vi "ClientAsig.vi"() -> ()   [LabVIEW 2021]
uses:
  <vilib>/Utility/file.llb/Write Delimited Spreadsheet (string).vi
panel:
  in  "login database":string[][](table)
  in  "Tab Control":T1(tab)
  in  "register":bool
  in  "login":bool
  in  "Password":string
  in  "Username":string
  in  "Front door":bool
  in  "On / off":bool
  in  "LR light 4":bool
  in  "LR light 3":bool
  in  "LR light 2":bool
  in  "LR light1":bool
  in  "LR curtain":dbl(knob) scale=0.0..100.0
  in  "aircorn temp":dbl(knob) scale=16.0..28.0
  in  "mb light 2":bool
  in  "mb light 1":bool
  in  "mb door":bool
  in  "bd light 1":bool
  in  "bd2 light 1":bool
  in  "bd2 light 2":bool
  in  "bd2 curtain 2":dbl(knob) scale=0.0..100.0
  in  "date&time":bool
  in  "balcony ct":dbl(knob) scale=0.0..100.0
  in  "balcony 1 light":bool
  in  "balcony light 1":bool
  in  "balcony light 2":bool
  in  "balcony light 3":bool
  in  "balcony1 ct":dbl(knob) scale=0.0..100.0
  in  "30 secs":bool
  in  "kc light 1":bool
  in  "kc light 2":bool
  in  "kc light 3":bool
  in  "Forward Button":bool
  in  "Back Button":bool
  in  "Pause Button":bool
  in  "mute":bool
  in  "volume":dbl(knob) scale=0.0..100.0
  in  "tv button3":bool
  in  "tv on":bool
  in  "tv off":bool
  in  "tv button 2":bool
  in  "tv button1":bool
  in  "forward":bool
  in  "back":bool
  in  "Refresh":bool
  in  "open":bool
  in  "website":string(combo)
  # "Welcome home"
  # "click other room to view other control"
  # "Living Room"
  # "lightning"
  # "aircorn"
  # "Curtain"
  # "master bedroom"
  # "lightning"
  # "door"
  # "bedroom 1"
  # "bedroom 2"
  # "lightning"
  # "curtain"
  # "balcony"
  # "lightning"
  # "curtain"
  # "Kitchen"
  # "timer"
  # "remote control TV"
  # "web broswer"
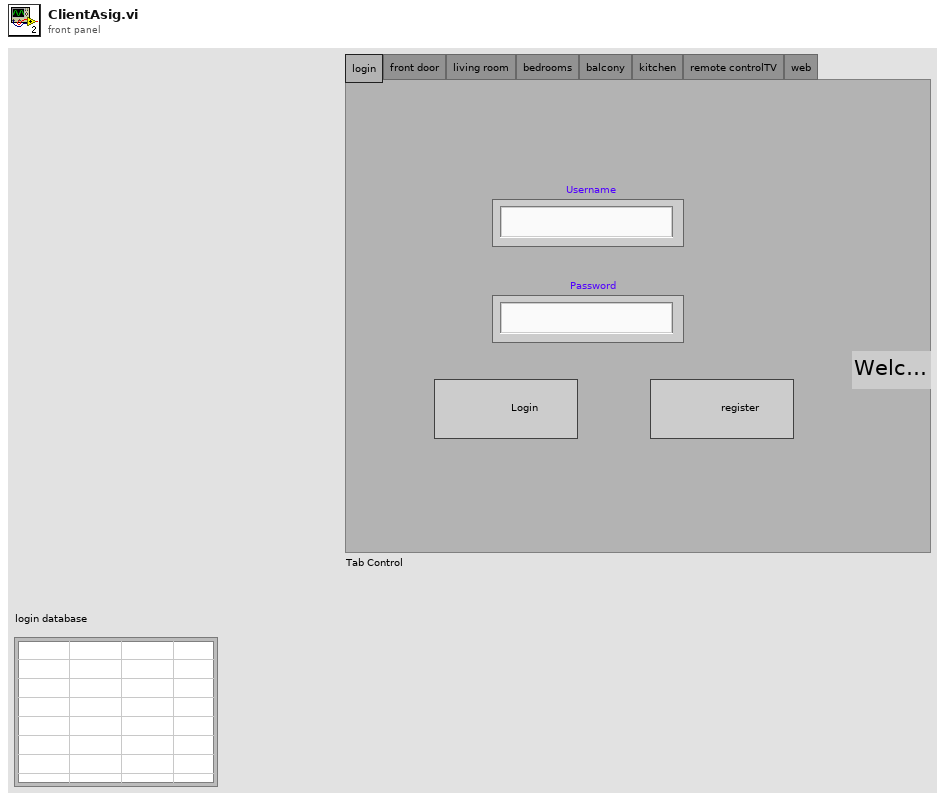
[diagram p1: front panel]
types:
  T1 = enum32{"login", "front door", "living room", "bedrooms", "balcony", "kitchen", "remote controlTV", "web"}
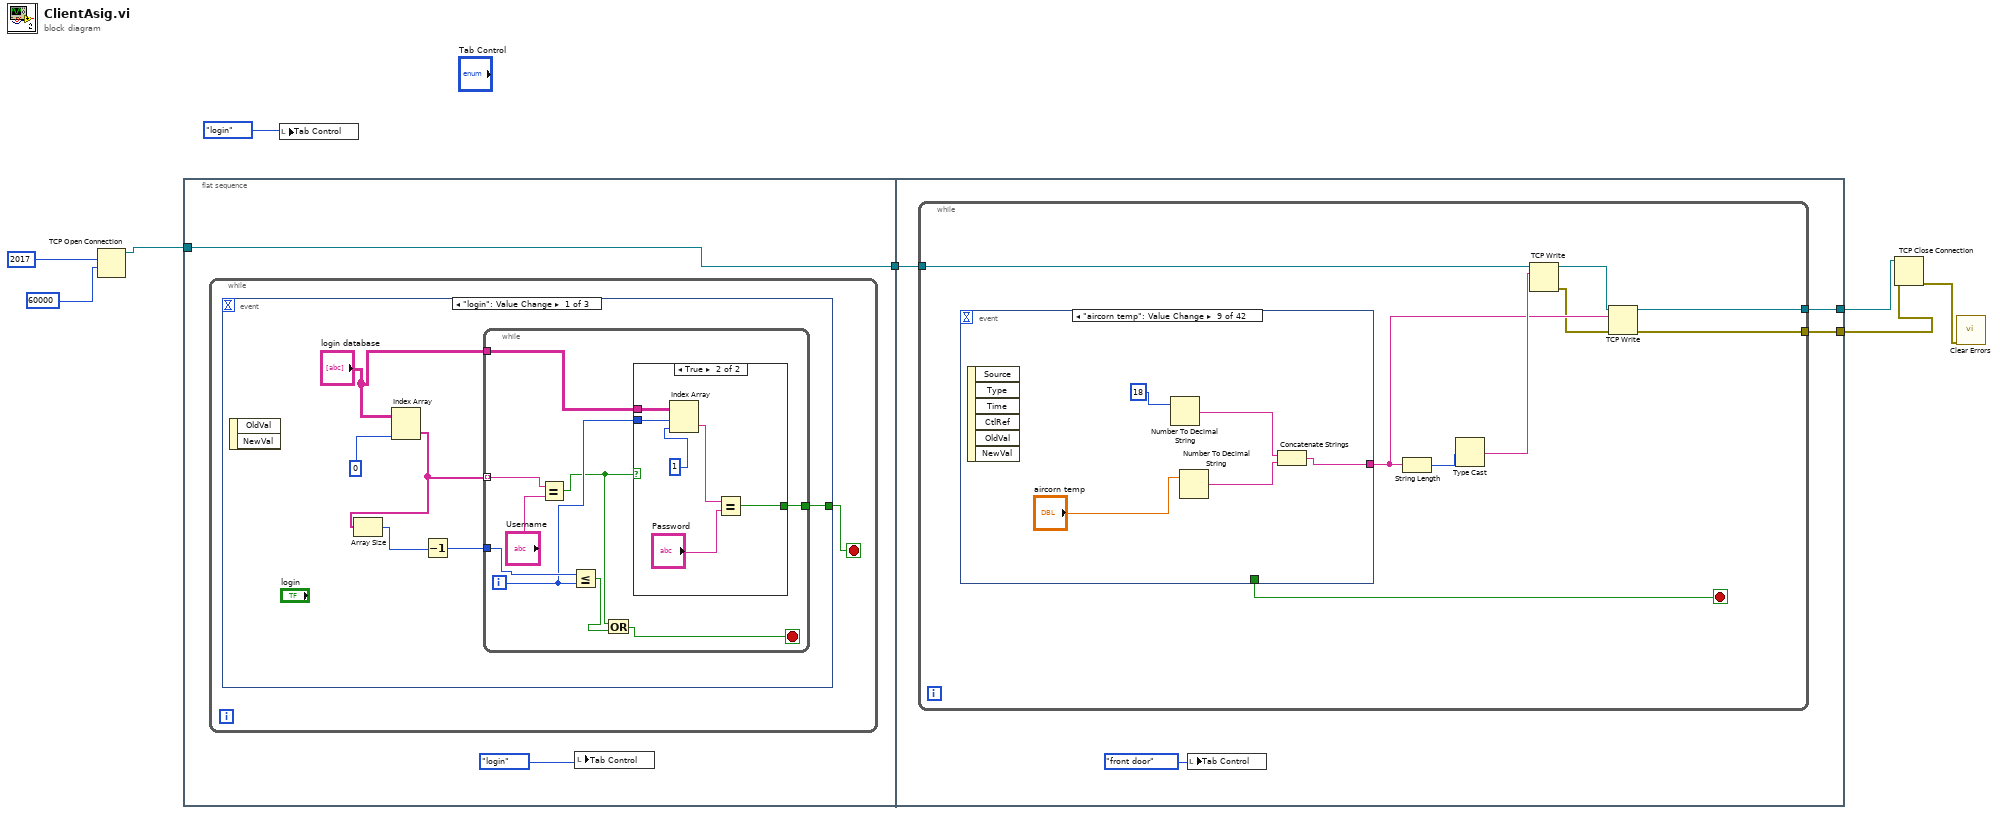
[diagram p0: block diagram]
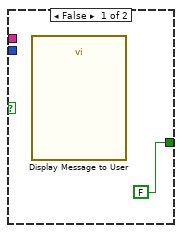
[diagram p2: hidden frame]
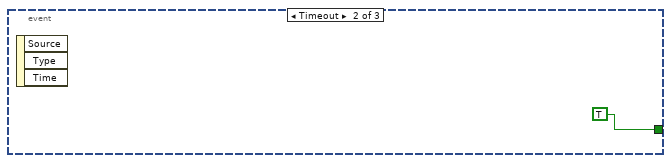
[diagram p3: hidden frame]
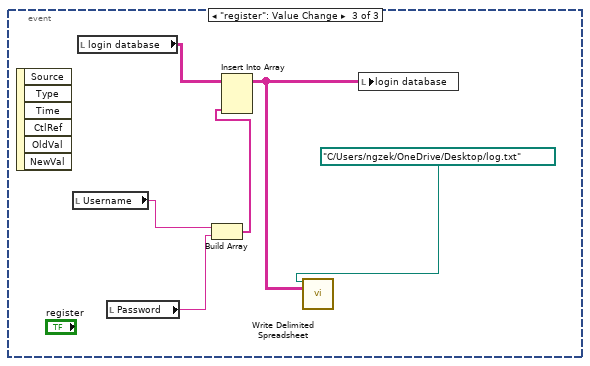
[diagram p4: hidden frame]
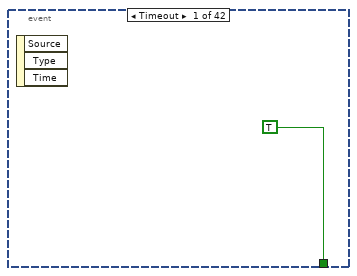
[diagram p5: hidden frame]
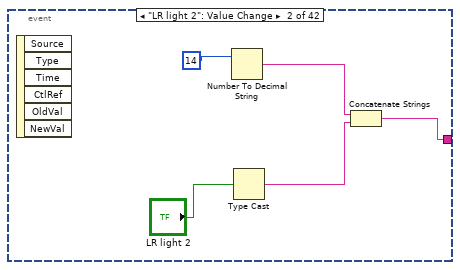
[diagram p6: hidden frame]
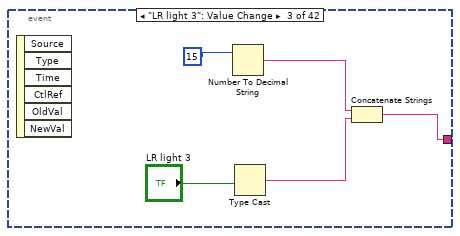
[diagram p7: hidden frame]
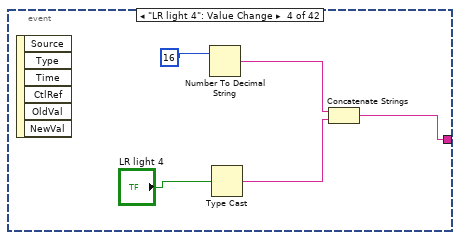
[diagram p8: hidden frame]
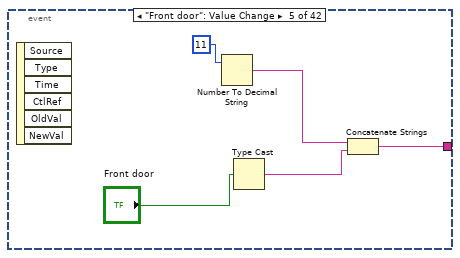
[diagram p9: hidden frame]
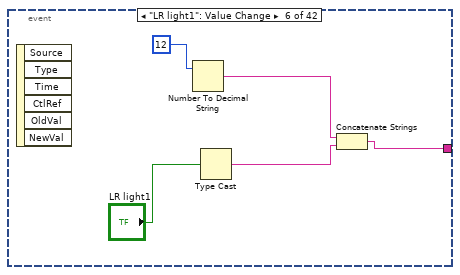
[diagram p10: hidden frame]
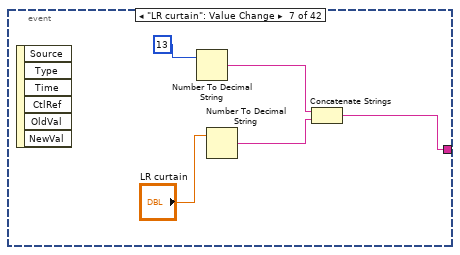
[diagram p11: hidden frame]
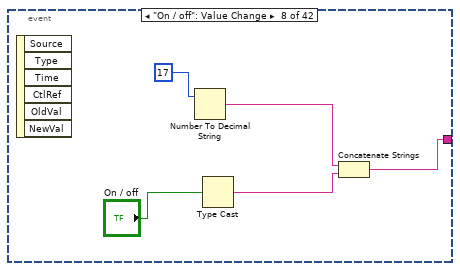
[diagram p12: hidden frame]
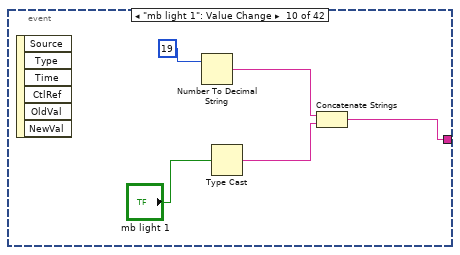
[diagram p13: hidden frame]
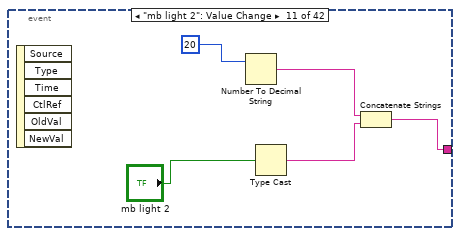
[diagram p14: hidden frame]
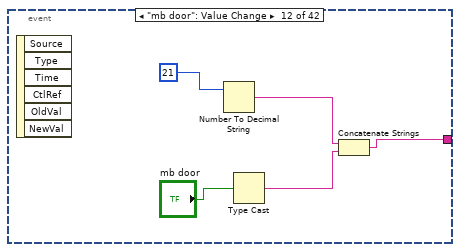
[diagram p15: hidden frame]
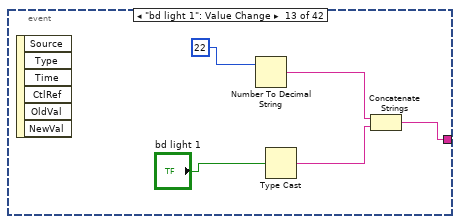
[diagram p16: hidden frame]
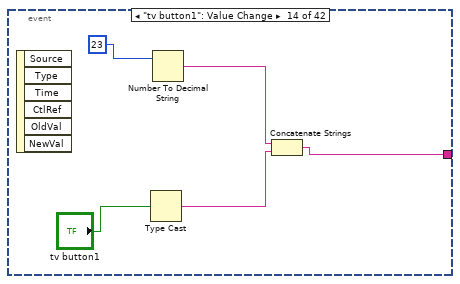
[diagram p17: hidden frame]
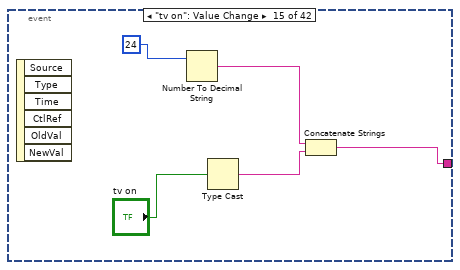
[diagram p18: hidden frame]
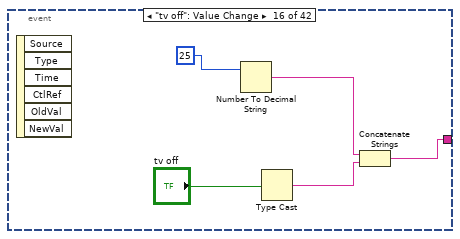
[diagram p19: hidden frame]
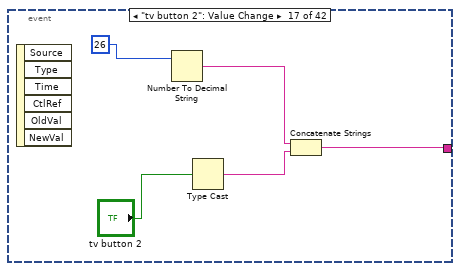
[diagram p20: hidden frame]
diagram:
  n1 = TCP Open Connection(remote port or service name=2017, timeout ms (60000)=60000) -> (connection ID=w4:refnum<k5>)  [unwired: 3 in, 1 out]
  n2 = flat-sequence {
    tunnel: [w10] -> w5
    tunnel: w4 -> [w10]
    tunnel: w5 -> [w44]
    tunnel: [w43] -> w3
    tunnel: [w42] -> w2
    frame #0 {
      n3 = while {
        stop <- w11 stop-if-true
        n4 = event shown="[0] \"login\": Value Change" {
          selector: _ -> [_ _ _]
          dyn-events: _ -> [_ _ _]
          timeout: _ -> [_ _ _]
          tunnel: [w12 TRUE _] -> w11
          event "login": Value Change {
            n5 = event-data() -> ()  [unwired: 1 in, 2 out]
            n6 = Index Array "Index Array"(array="login database", index (col)=0) -> (element=w14:string[])  [unwired: 1 in]
            n7 = Array Size(array=w14) -> (size(s)=w16:i32)
            n8 = Decrement(x=w16) -> (x-1=w13:i32)
            n9 = while {
              tunnel: "login database" -> [w26]
              tunnel: w14 -> [w25] mode=indexing
              tunnel: w13 -> [w23]
              tunnel: [w18] -> w12
              i -> [w22]
              stop <- w19 stop-if-true
              n10 = Equal?(x=w25, y="Username") -> (x = y?=w21:bool)
              n11 = Less Or Equal?(x=w23, y=w22) -> (x <= y?=w20:bool)
              n12 = Or(x=w21, y=w20) -> (x .or. y?=w19:bool)
              n13 = case shown="True" w21 {
                tunnel: w26 -> [_ w33]
                tunnel: w22 -> [_ w31]
                tunnel: [FALSE w28] -> w18
                frame False {
                  n14 = call "Display Message to User"() -> ()  [unwired: 10 in, 2 out]
                }
                frame True {
                  n15 = Index Array "Index Array"(array=w33, index (row)=w31, index (col)=1) -> (element=w30:string)
                  n16 = Equal?(x=w30, y="Password") -> (x = y?=w28:bool)
                }
              }
            }
          }
          event Timeout {
            n17 = event-data() -> ()  [unwired: 1 in, 3 out]
          }
          event "register": Value Change {
            n18 = event-data() -> ()  [unwired: 1 in, 6 out]
            n19 = local read "Username"() -> (w39:string)
            n20 = local read "login database"() -> (w40:string[][])
            n21 = local read "Password"() -> (w38:string)
            n22 = Build Array "Build Array"(w39, w38) -> (w37:string[])
            n23 = Insert Into Array "Insert Into Array"(array=w40, new element=w37) -> (w36:string[][])  [unwired: 2 in]
            n24 = call-poly <vilib>:"Write Delimited Spreadsheet.vi"("file path (dialog if empty)"=path "C:/Users/ngzek/OneDrive/Desktop/log.txt", "2D data"=w36) -> ()  [unwired: 12 in, 2 out]
            n25 = local write "login database"(w36) -> ()
          }
        }
      }
      n26 = local write "Tab Control"(enum32{"login", "front door"}."login" ("Tab Control")) -> ()
    }
    frame #1 {
      n27 = while {
        tunnel: w44 -> [w53]
        tunnel: [w49] -> w42
        tunnel: [w45] -> w43
        stop <- w48 stop-if-true
        n28 = event shown="[8] \"aircorn temp\": Value Change" {
          selector: _ -> [_ _ _ _ _ _ _ _ _ _ _ _ _ _ _ _ _ _ _ _ _ _ _ _ _ _ _ _ _ _ _ _ _ _ _ _ _ _ _ _ _ _]
          dyn-events: _ -> [_ _ _ _ _ _ _ _ _ _ _ _ _ _ _ _ _ _ _ _ _ _ _ _ _ _ _ _ _ _ _ _ _ _ _ _ _ _ _ _ _ _]
          timeout: _ -> [_ _ _ _ _ _ _ _ _ _ _ _ _ _ _ _ _ _ _ _ _ _ _ _ _ _ _ _ _ _ _ _ _ _ _ _ _ _ _ _ _ _]
          tunnel: [_ w55 w60 w65 w70 w75 w80 w85 w90 w97 w100 w105 w110 w115 w120 w125 w130 w135 w140 w145 w150 w155 w160 w165 w170 w175 w180 w185 w190 w195 w200 w205 w210 w215 w220 w225 w230 w234 w239 w244 w249 w254] -> w47
          tunnel: [TRUE _ _ _ _ _ _ _ _ _ _ _ _ _ _ _ _ _ _ _ _ _ _ _ _ _ _ _ _ _ _ _ _ _ _ _ _ _ _ _ _ _] -> w48
          event Timeout {
            n29 = event-data() -> ()  [unwired: 1 in, 3 out]
          }
          event "LR light 2": Value Change {
            n30 = event-data() -> ()  [unwired: 1 in, 6 out]
            n31 = Number To Decimal String(number=14) -> (decimal integer string=w56:string)  [unwired: 1 in]
            n32 = Type Cast(x="LR light 2") -> (*(type *) &x=w57:string)  [unwired: 1 in]
            n33 = Concatenate Strings(w56, w57) -> (w55:string)
          }
          event "LR light 3": Value Change {
            n34 = event-data() -> ()  [unwired: 1 in, 6 out]
            n35 = Number To Decimal String(number=15) -> (decimal integer string=w62:string)  [unwired: 1 in]
            n36 = Type Cast(x="LR light 3") -> (*(type *) &x=w63:string)  [unwired: 1 in]
            n37 = Concatenate Strings(w62, w63) -> (w60:string)
          }
          event "LR light 4": Value Change {
            n38 = event-data() -> ()  [unwired: 1 in, 6 out]
            n39 = Number To Decimal String(number=16) -> (decimal integer string=w68:string)  [unwired: 1 in]
            n40 = Type Cast(x="LR light 4") -> (*(type *) &x=w67:string)  [unwired: 1 in]
            n41 = Concatenate Strings(w68, w67) -> (w65:string)
          }
          event "Front door": Value Change {
            n42 = event-data() -> ()  [unwired: 1 in, 6 out]
            n43 = Number To Decimal String(number=11) -> (decimal integer string=w73:string)  [unwired: 1 in]
            n44 = Type Cast(x="Front door") -> (*(type *) &x=w71:string)  [unwired: 1 in]
            n45 = Concatenate Strings "Concatenate Strings"(w73, w71) -> (w70:string)
          }
          event "LR light1": Value Change {
            n46 = event-data() -> ()  [unwired: 1 in, 6 out]
            n47 = Number To Decimal String(number=12) -> (decimal integer string=w78:string)  [unwired: 1 in]
            n48 = Type Cast(x="LR light1") -> (*(type *) &x=w76:string)  [unwired: 1 in]
            n49 = Concatenate Strings(w78, w76) -> (w75:string)
          }
          event "LR curtain": Value Change {
            n50 = event-data() -> ()  [unwired: 1 in, 6 out]
            n51 = Number To Decimal String(number=13) -> (decimal integer string=w82:string)  [unwired: 1 in]
            n52 = Number To Decimal String(number="LR curtain") -> (decimal integer string=w81:string)  [unwired: 1 in]
            n53 = Concatenate Strings(w82, w81) -> (w80:string)
          }
          event "On / off": Value Change {
            n54 = event-data() -> ()  [unwired: 1 in, 6 out]
            n55 = Number To Decimal String(number=17) -> (decimal integer string=w89:string)  [unwired: 1 in]
            n56 = Type Cast(x="On / off") -> (*(type *) &x=w88:string)  [unwired: 1 in]
            n57 = Concatenate Strings(w89, w88) -> (w85:string)
          }
          event "aircorn temp": Value Change {
            n58 = event-data() -> ()  [unwired: 1 in, 6 out]
            n59 = Number To Decimal String(number=18) -> (decimal integer string=w93:string)  [unwired: 1 in]
            n60 = Number To Decimal String(number="aircorn temp") -> (decimal integer string=w92:string)  [unwired: 1 in]
            n61 = Concatenate Strings(w93, w92) -> (w90:string)
          }
          event "mb light 1": Value Change {
            n62 = event-data() -> ()  [unwired: 1 in, 6 out]
            n63 = Number To Decimal String(number=19) -> (decimal integer string=w99:string)  [unwired: 1 in]
            n64 = Type Cast(x="mb light 1") -> (*(type *) &x=w95:string)  [unwired: 1 in]
            n65 = Concatenate Strings(w99, w95) -> (w97:string)
          }
          event "mb light 2": Value Change {
            n66 = event-data() -> ()  [unwired: 1 in, 6 out]
            n67 = Number To Decimal String(number=20) -> (decimal integer string=w104:string)  [unwired: 1 in]
            n68 = Type Cast(x="mb light 2") -> (*(type *) &x=w103:string)  [unwired: 1 in]
            n69 = Concatenate Strings(w104, w103) -> (w100:string)
          }
          event "mb door": Value Change {
            n70 = event-data() -> ()  [unwired: 1 in, 6 out]
            n71 = Number To Decimal String(number=21) -> (decimal integer string=w109:string)  [unwired: 1 in]
            n72 = Type Cast(x="mb door") -> (*(type *) &x=w108:string)  [unwired: 1 in]
            n73 = Concatenate Strings(w109, w108) -> (w105:string)
          }
          event "bd light 1": Value Change {
            n74 = event-data() -> ()  [unwired: 1 in, 6 out]
            n75 = Number To Decimal String(number=22) -> (decimal integer string=w114:string)  [unwired: 1 in]
            n76 = Type Cast(x="bd light 1") -> (*(type *) &x=w113:string)  [unwired: 1 in]
            n77 = Concatenate Strings(w114, w113) -> (w110:string)
          }
          event "tv button1": Value Change {
            n78 = event-data() -> ()  [unwired: 1 in, 6 out]
            n79 = Type Cast(x="tv button1") -> (*(type *) &x=w117:string)  [unwired: 1 in]
            n80 = Number To Decimal String(number=23) -> (decimal integer string=w116:string)  [unwired: 1 in]
            n81 = Concatenate Strings(w116, w117) -> (w115:string)
          }
          event "tv on": Value Change {
            n82 = event-data() -> ()  [unwired: 1 in, 6 out]
            n83 = Number To Decimal String(number=24) -> (decimal integer string=w124:string)  [unwired: 1 in]
            n84 = Type Cast(x="tv on") -> (*(type *) &x=w121:string)  [unwired: 1 in]
            n85 = Concatenate Strings(w124, w121) -> (w120:string)
          }
          event "tv off": Value Change {
            n86 = event-data() -> ()  [unwired: 1 in, 6 out]
            n87 = Number To Decimal String(number=25) -> (decimal integer string=w129:string)  [unwired: 1 in]
            n88 = Type Cast(x="tv off") -> (*(type *) &x=w128:string)  [unwired: 1 in]
            n89 = Concatenate Strings(w129, w128) -> (w125:string)
          }
          event "tv button 2": Value Change {
            n90 = event-data() -> ()  [unwired: 1 in, 6 out]
            n91 = Number To Decimal String(number=26) -> (decimal integer string=w134:string)  [unwired: 1 in]
            n92 = Type Cast(x="tv button 2") -> (*(type *) &x=w133:string)  [unwired: 1 in]
            n93 = Concatenate Strings(w134, w133) -> (w130:string)
          }
          event "tv button3": Value Change {
            n94 = event-data() -> ()  [unwired: 1 in, 6 out]
            n95 = Number To Decimal String(number=27) -> (decimal integer string=w139:string)  [unwired: 1 in]
            n96 = Type Cast(x="tv button3") -> (*(type *) &x=w138:string)  [unwired: 1 in]
            n97 = Concatenate Strings(w139, w138) -> (w135:string)
          }
          event "volume": Value Change {
            n98 = event-data() -> ()  [unwired: 1 in, 6 out]
            n99 = Number To Decimal String(number=28) -> (decimal integer string=w144:string)  [unwired: 1 in]
            n100 = Number To Decimal String(number="volume") -> (decimal integer string=w143:string)  [unwired: 1 in]
            n101 = Concatenate Strings(w144, w143) -> (w140:string)
          }
          event "mute": Value Change {
            n102 = event-data() -> ()  [unwired: 1 in, 6 out]
            n103 = Number To Decimal String(number=29) -> (decimal integer string=w149:string)  [unwired: 1 in]
            n104 = Type Cast(x="mute") -> (*(type *) &x=w148:string)  [unwired: 1 in]
            n105 = Concatenate Strings(w149, w148) -> (w145:string)
          }
          event "Pause Button": Value Change {
            n106 = event-data() -> ()  [unwired: 1 in, 6 out]
            n107 = Number To Decimal String(number=30) -> (decimal integer string=w154:string)  [unwired: 1 in]
            n108 = Type Cast(x="Pause Button") -> (*(type *) &x=w151:string)  [unwired: 1 in]
            n109 = Concatenate Strings(w154, w151) -> (w150:string)
          }
          event "Forward Button": Value Change {
            n110 = event-data() -> ()  [unwired: 1 in, 6 out]
            n111 = Number To Decimal String(number=31) -> (decimal integer string=w159:string)  [unwired: 1 in]
            n112 = Type Cast(x="Forward Button") -> (*(type *) &x=w158:string)  [unwired: 1 in]
            n113 = Concatenate Strings(w159, w158) -> (w155:string)
          }
          event "Back Button": Value Change {
            n114 = event-data() -> ()  [unwired: 1 in, 6 out]
            n115 = Number To Decimal String(number=32) -> (decimal integer string=w163:string)  [unwired: 1 in]
            n116 = Type Cast(x="Back Button") -> (*(type *) &x=w162:string)  [unwired: 1 in]
            n117 = Concatenate Strings(w163, w162) -> (w160:string)
          }
          event "bd2 light 1": Value Change {
            n118 = event-data() -> ()  [unwired: 1 in, 6 out]
            n119 = Number To Decimal String(number=33) -> (decimal integer string=w169:string)  [unwired: 1 in]
            n120 = Type Cast(x="bd2 light 1") -> (*(type *) &x=w168:string)  [unwired: 1 in]
            n121 = Concatenate Strings(w169, w168) -> (w165:string)
          }
          event "bd2 light 2": Value Change {
            n122 = event-data() -> ()  [unwired: 1 in, 6 out]
            n123 = Number To Decimal String(number=34) -> (decimal integer string=w174:string)  [unwired: 1 in]
            n124 = Type Cast(x="bd2 light 2") -> (*(type *) &x=w173:string)  [unwired: 1 in]
            n125 = Concatenate Strings(w174, w173) -> (w170:string)
          }
          event "bd2 curtain 2": Value Change {
            n126 = event-data() -> ()  [unwired: 1 in, 6 out]
            n127 = Number To Decimal String(number=35) -> (decimal integer string=w179:string)  [unwired: 1 in]
            n128 = Number To Decimal String(number="bd2 curtain 2") -> (decimal integer string=w178:string)  [unwired: 1 in]
            n129 = Concatenate Strings(w179, w178) -> (w175:string)
          }
          event "balcony light 1": Value Change {
            n130 = event-data() -> ()  [unwired: 1 in, 6 out]
            n131 = Number To Decimal String(number=36) -> (decimal integer string=w183:string)  [unwired: 1 in]
            n132 = Type Cast(x="balcony light 1") -> (*(type *) &x=w182:string)  [unwired: 1 in]
            n133 = Concatenate Strings(w183, w182) -> (w180:string)
          }
          event "balcony light 2": Value Change {
            n134 = event-data() -> ()  [unwired: 1 in, 6 out]
            n135 = Number To Decimal String(number=37) -> (decimal integer string=w189:string)  [unwired: 1 in]
            n136 = Type Cast(x="balcony light 2") -> (*(type *) &x=w188:string)  [unwired: 1 in]
            n137 = Concatenate Strings(w189, w188) -> (w185:string)
          }
          event "balcony light 3": Value Change {
            n138 = event-data() -> ()  [unwired: 1 in, 6 out]
            n139 = Number To Decimal String(number=38) -> (decimal integer string=w194:string)  [unwired: 1 in]
            n140 = Type Cast(x="balcony light 3") -> (*(type *) &x=w193:string)  [unwired: 1 in]
            n141 = Concatenate Strings(w194, w193) -> (w190:string)
          }
          event "balcony 1 light": Value Change {
            n142 = event-data() -> ()  [unwired: 1 in, 6 out]
            n143 = Number To Decimal String(number=39) -> (decimal integer string=w199:string)  [unwired: 1 in]
            n144 = Type Cast(x="balcony 1 light") -> (*(type *) &x=w198:string)  [unwired: 1 in]
            n145 = Concatenate Strings(w199, w198) -> (w195:string)
          }
          event "kc light 1": Value Change {
            n146 = event-data() -> ()  [unwired: 1 in, 6 out]
            n147 = Number To Decimal String(number=40) -> (decimal integer string=w204:string)  [unwired: 1 in]
            n148 = Type Cast(x="kc light 1") -> (*(type *) &x=w203:string)  [unwired: 1 in]
            n149 = Concatenate Strings(w204, w203) -> (w200:string)
          }
          event "kc light 2": Value Change {
            n150 = event-data() -> ()  [unwired: 1 in, 6 out]
            n151 = Number To Decimal String(number=41) -> (decimal integer string=w208:string)  [unwired: 1 in]
            n152 = Type Cast(x="kc light 2") -> (*(type *) &x=w209:string)  [unwired: 1 in]
            n153 = Concatenate Strings(w208, w209) -> (w205:string)
          }
          event "kc light 3": Value Change {
            n154 = event-data() -> ()  [unwired: 1 in, 6 out]
            n155 = Number To Decimal String(number=42) -> (decimal integer string=w213:string)  [unwired: 1 in]
            n156 = Type Cast(x="kc light 3") -> (*(type *) &x=w212:string)  [unwired: 1 in]
            n157 = Concatenate Strings(w213, w212) -> (w210:string)
          }
          event "date&time": Value Change {
            n158 = event-data() -> ()  [unwired: 1 in, 6 out]
            n159 = Number To Decimal String(number=43) -> (decimal integer string=w219:string)  [unwired: 1 in]
            n160 = Type Cast(x="date&time") -> (*(type *) &x=w216:string)  [unwired: 1 in]
            n161 = Concatenate Strings "Concatenate Strings"(w219, w216) -> (w215:string)
          }
          event "30 secs": Value Change {
            n162 = event-data() -> ()  [unwired: 1 in, 6 out]
            n163 = Number To Decimal String(number=44) -> (decimal integer string=w224:string)  [unwired: 1 in]
            n164 = Type Cast(x="30 secs") -> (*(type *) &x=w223:string)  [unwired: 1 in]
            n165 = Concatenate Strings(w224, w223) -> (w220:string)
          }
          event "open": Value Change {
            n166 = event-data() -> ()  [unwired: 1 in, 6 out]
            n167 = Number To Decimal String(number=45) -> (decimal integer string=w229:string)  [unwired: 1 in]
            n168 = Type Cast(x="open") -> (*(type *) &x=w228:string)  [unwired: 1 in]
            n169 = Concatenate Strings(w229, w228) -> (w225:string)
          }
          event "website": Value Change {
            n170 = event-data() -> ()  [unwired: 1 in, 6 out]
            n171 = Number To Decimal String(number=46) -> (decimal integer string=w233:string)  [unwired: 1 in]
            n172 = Concatenate Strings(w233, "website") -> (w230:string)
          }
          event "Refresh": Value Change {
            n173 = event-data() -> ()  [unwired: 1 in, 6 out]
            n174 = Type Cast(x="Refresh") -> (*(type *) &x=w235:string)  [unwired: 1 in]
            n175 = Number To Decimal String(number=47) -> (decimal integer string=w238:string)  [unwired: 1 in]
            n176 = Concatenate Strings(w238, w235) -> (w234:string)
          }
          event "back": Value Change {
            n177 = event-data() -> ()  [unwired: 1 in, 6 out]
            n178 = Type Cast(x="back") -> (*(type *) &x=w242:string)  [unwired: 1 in]
            n179 = Number To Decimal String(number=48) -> (decimal integer string=w243:string)  [unwired: 1 in]
            n180 = Concatenate Strings(w243, w242) -> (w239:string)
          }
          event "forward": Value Change {
            n181 = event-data() -> ()  [unwired: 1 in, 6 out]
            n182 = Type Cast(x="forward") -> (*(type *) &x=w248:string)  [unwired: 1 in]
            n183 = Number To Decimal String(number=49) -> (decimal integer string=w247:string)  [unwired: 1 in]
            n184 = Concatenate Strings(w247, w248) -> (w244:string)
          }
          event "balcony ct": Value Change {
            n185 = event-data() -> ()  [unwired: 1 in, 6 out]
            n186 = Number To Decimal String(number=50) -> (decimal integer string=w253:string)  [unwired: 1 in]
            n187 = Number To Decimal String(number="balcony ct") -> (decimal integer string=w252:string)  [unwired: 1 in]
            n188 = Concatenate Strings(w253, w252) -> (w249:string)
          }
          event "balcony1 ct": Value Change {
            n189 = event-data() -> ()  [unwired: 1 in, 6 out]
            n190 = Number To Decimal String(number=51) -> (decimal integer string=w258:string)  [unwired: 1 in]
            n191 = Number To Decimal String(number="balcony1 ct") -> (decimal integer string=w257:string)  [unwired: 1 in]
            n192 = Concatenate Strings(w258, w257) -> (w254:string)
          }
        }
        n193 = String Length(string=w47) -> (length=w52:i32)
        n194 = Type Cast(x=w52) -> (*(type *) &x=w51:string)  [unwired: 1 in]
        n195 = TCP Write(connection ID=w53, data in=w51) -> (connection ID out=w50:refnum<k5>, error out=w46:errorcluster)  [unwired: 2 in, 1 out]
        n196 = TCP Write(connection ID=w50, data in=w47, error in (no error)=w46) -> (connection ID out=w49:refnum<k5>, error out=w45:errorcluster)  [unwired: 1 in, 1 out]
      }
      n197 = local write "Tab Control"(enum32{"login", "front door"}."front door" ("Tab Control")) -> ()
    }
  }
  n198 = local write "Tab Control"(enum32{"login", "front door"}."login" ("Tab Control")) -> ()
  n199 = TCP Close Connection(connection ID=w2, error in (no error)=w3) -> (error out=w6:errorcluster)  [unwired: 1 in, 1 out]
  n200 = call <vilib>:"Clear Errors.vi"("error in (no error)"=w6) -> ()  [unwired: 5 in, 2 out]
